vi "Tool for Program after.vi"(8 "error in (no error)":errorcluster, 9 "Cmd In":string="$AGENT,52,FORMAT*5D", 10 "VISA resource name":refnum<visa-resource-name>="COM3", 11 "action":u16(ring) items=["ProjectName", "Name", "Initial", "Reset", "Format", "Program1", "Program2", "Scan"]) -> (0 "error out":errorcluster, 3 "receive string":string)   [LabVIEW 2019]
panel:
  in  "Boolean":bool
  out "read string":string
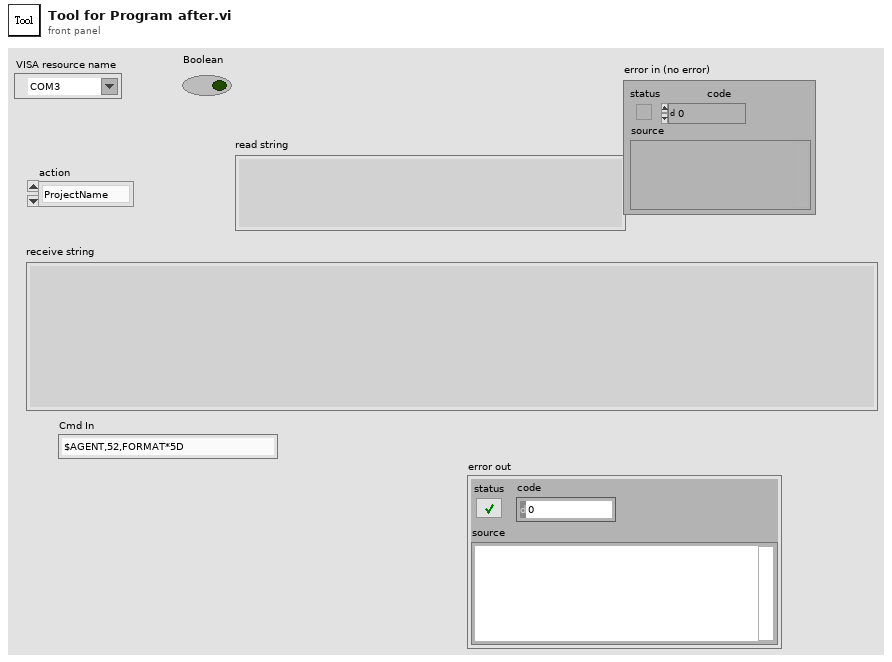
[diagram p1: front panel]
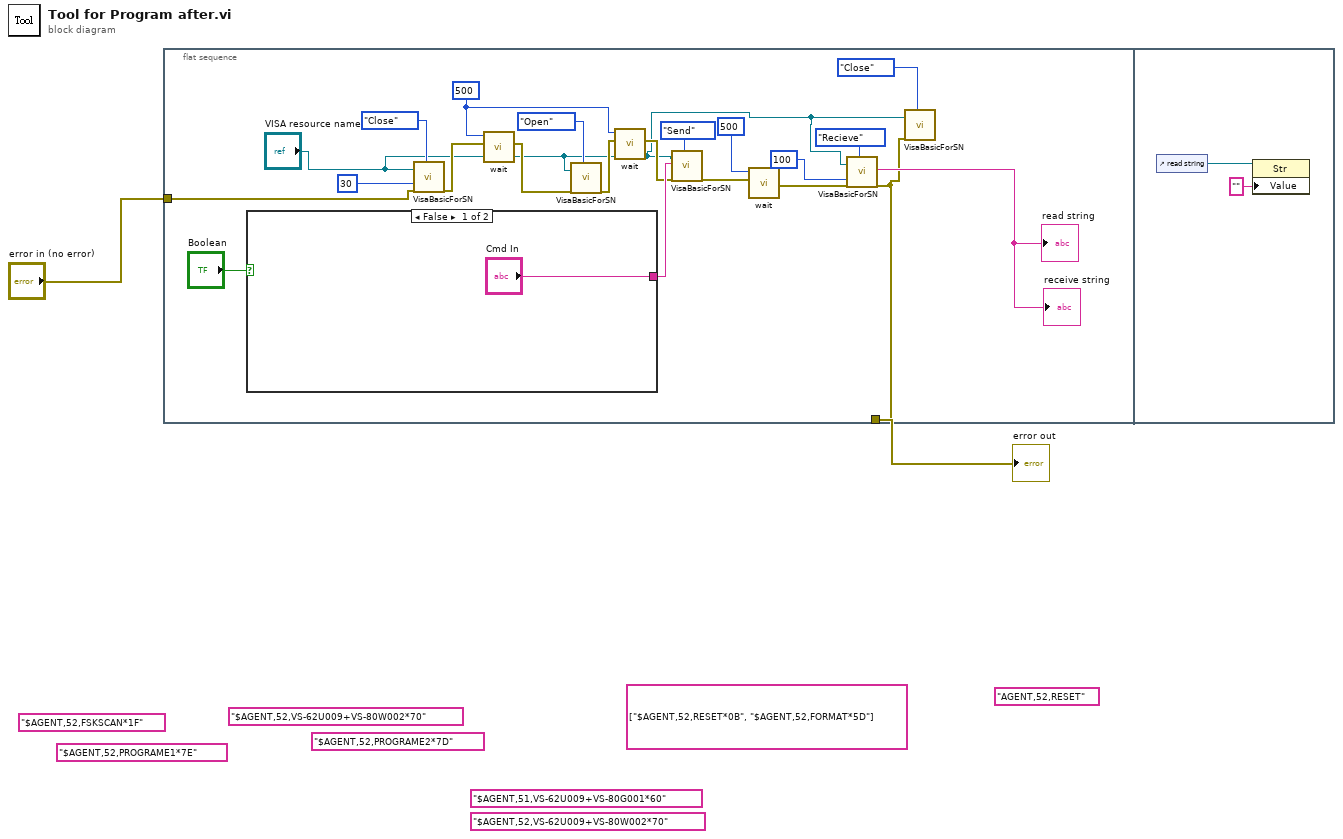
[diagram p0: block diagram]
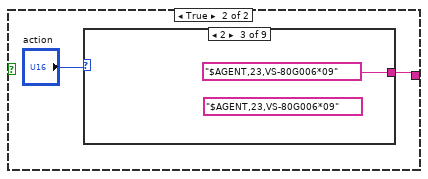
[diagram p2: hidden frame]
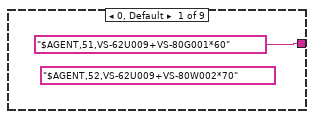
[diagram p3: hidden frame]
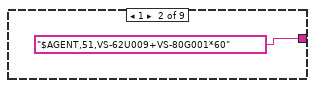
[diagram p4: hidden frame]
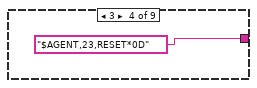
[diagram p5: hidden frame]
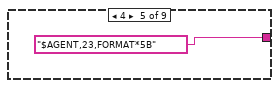
[diagram p6: hidden frame]
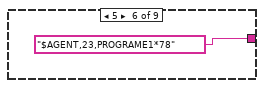
[diagram p7: hidden frame]
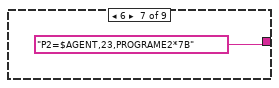
[diagram p8: hidden frame]
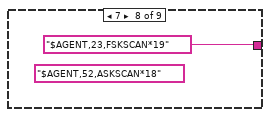
[diagram p9: hidden frame]
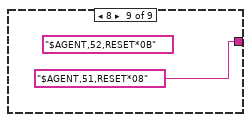
[diagram p10: hidden frame]
diagram:
  (unwired) "$AGENT,52,FSKSCAN*1F" ("Cmd 2")
  (unwired) "$AGENT,52,PROGRAME2*7D" ("Cmd 2")
  (unwired) "$AGENT,52,PROGRAME1*7E" ("Cmd 2")
  (unwired) "$AGENT,51,VS-62U009+VS-80G001*60" ("Cmd 2")
  (unwired) "$AGENT,52,VS-62U009+VS-80W002*70" ("Cmd 2")
  (unwired) "AGENT,52,RESET"
  (unwired) "$AGENT,52,VS-62U009+VS-80W002*70" ("Cmd 2")
  (unwired) string[] ["$AGENT,52,RESET*0B", "$AGENT,52,FORMAT*5D"]
  n1 = flat-sequence {
    tunnel: [w5] -> w2
    tunnel: "error in (no error)" -> [w13]
    frame #0 {
      w6 = u32 500 ("wait(ms)")
      n2 = case shown="False" "Boolean" {
        tunnel: ["Cmd In" w25] -> w12
        frame False {
        }
        frame True {
          n3 = case shown="2" "action" {
            tunnel: ["$AGENT,51,VS-62U009+VS-80G001*60" ("Cmd 2") "$AGENT,51,VS-62U009+VS-80G001*60" ("Cmd 2") "$AGENT,23,VS-80G006*09" ("Cmd 2") "$AGENT,23,RESET*0D" ("Cmd 2") "$AGENT,23,FORMAT*5B" ("Cmd 2") "$AGENT,23,PROGRAME1*78" ("Cmd 2") "P2=$AGENT,23,PROGRAME2*7B" ("Cmd 2") "$AGENT,23,FSKSCAN*19" ("Cmd 2") "$AGENT,51,RESET*08" ("Cmd 2")] -> w25
            frame 0, Default {
              (unwired) "$AGENT,52,VS-62U009+VS-80W002*70" ("Cmd 2")
            }
            frame 1 {
            }
            frame 2 {
              (unwired) "$AGENT,23,VS-80G006*09" ("Cmd 2")
            }
            frame 3 {
            }
            frame 4 {
            }
            frame 5 {
            }
            frame 6 {
            }
            frame 7 {
              (unwired) "$AGENT,52,ASKSCAN*18" ("Cmd 2")
            }
            frame 8 {
              (unwired) "$AGENT,52,RESET*0B" ("Cmd 2")
            }
          }
        }
      }
      n4 = call "VisaBasicForSN.vi"("VISA resource name"="VISA resource name", "Time(0.1)"=30, "error in (no error)"=w13, "VisaAction"=enum16{"Open", "Send", "Recieve", "Close"}."Close") -> ("error out"=w10:errorcluster)  [unwired: 14 in, 1 out]
      n5 = call "wait.vi"("error in"=w10, "wait(ms)"=w6) -> ("error out"=w9:errorcluster)  [unwired: 9 in]
      n6 = call "VisaBasicForSN.vi"("VISA resource name"="VISA resource name", "error in (no error)"=w9, "VisaAction"=enum16{"Open", "Send", "Recieve", "Close"}."Open") -> ("error out"=w8:errorcluster)  [unwired: 15 in, 1 out]
      n7 = call "wait.vi"("error in"=w8, "wait(ms)"=w6) -> ("error out"=w7:errorcluster)  [unwired: 9 in]
      n8 = call "VisaBasicForSN.vi"("VISA resource name"="VISA resource name", "Cmd"=w12, "error in (no error)"=w7, "VisaAction"=enum16{"Open", "Send", "Recieve", "Close"}."Send") -> ("error out"=w15:errorcluster)  [unwired: 14 in, 1 out]
      n9 = call "wait.vi"("error in"=w15, "wait(ms)"=u32 500) -> ("error out"=w14:errorcluster)  [unwired: 9 in]
      n10 = call "VisaBasicForSN.vi"("VISA resource name"="VISA resource name", "Time(0.1)"=u32 100, "error in (no error)"=w14, "VisaAction"=enum16{"Open", "Send", "Recieve", "Close"}."Recieve") -> ("read string"=→"read string" →"receive string":string, "error out"=w5:errorcluster)  [unwired: 14 in]
      n11 = call "VisaBasicForSN.vi"("VISA resource name"="VISA resource name", "error in (no error)"=w5, "VisaAction"=enum16{"Open", "Send", "Recieve", "Close"}."Close") -> ()  [unwired: 15 in, 2 out]
    }
    frame #1 {
      n12 = control-ref of="read string"() -> (w37:refnum<vi>)
      n13 = property class="Str"(reference=w37, "Value"="") -> ()  [unwired: 1 in, 2 out]
    }
  }
  "error out" <- w2
